vi "fitting.vi"(0 "fitting type":dbl, 5 "2D data":dbl[][](array[numeric]), 7 "force guess?":bool, 9 "force guess value":dbl[](array[numeric])) -> (4 "best fit":dbl[][](array[numeric]), 6 "best fit parameters":dbl[](array[numeric]))   [LabVIEW 2013]
uses:
  <vilib>/gmath/NumericalOptimization/Nonlinear Curve Fit LM.vi
  <vilib>/gmath/NI_Gmath.lvlib
panel:
  out "number of function calls":i32 caption="函数调用次数"
  out "数组":i32[](array[numeric])
  out "输出数组":dbl[](array[numeric])
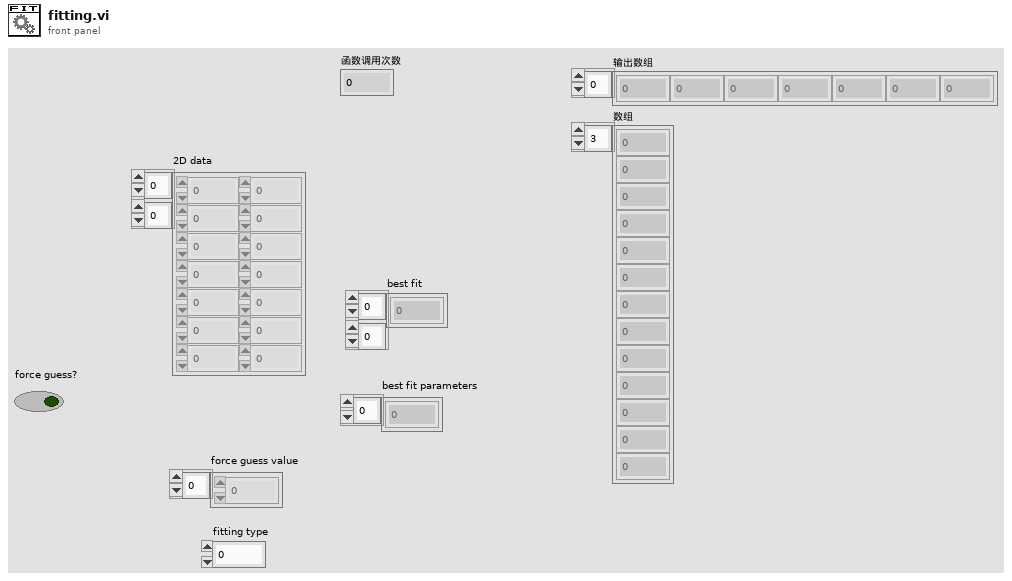
[diagram p1: front panel]
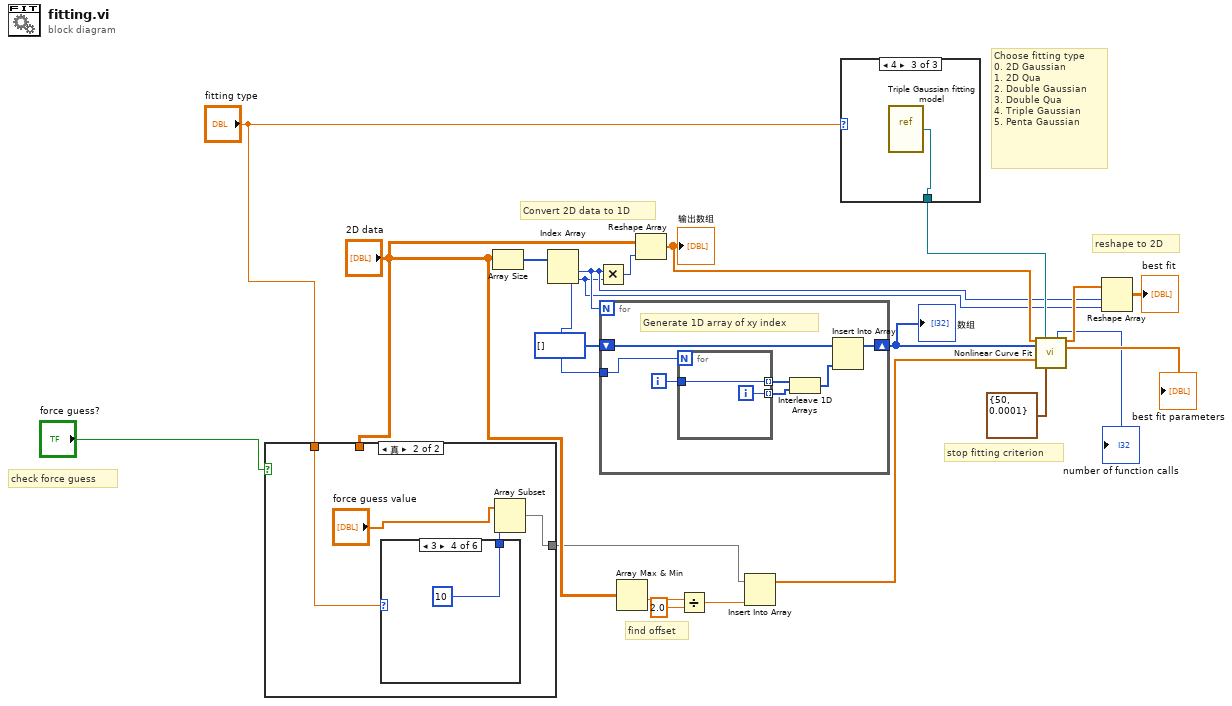
[diagram p0: block diagram]
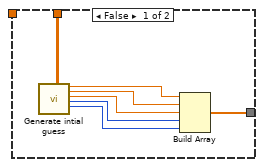
[diagram p2: hidden frame]
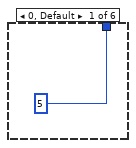
[diagram p3: hidden frame]
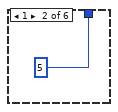
[diagram p4: hidden frame]
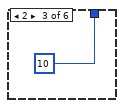
[diagram p5: hidden frame]
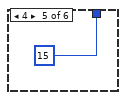
[diagram p6: hidden frame]
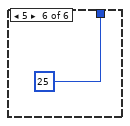
[diagram p7: hidden frame]
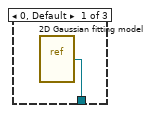
[diagram p8: hidden frame]
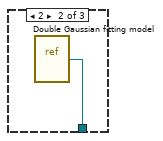
[diagram p9: hidden frame]
diagram:
  # "reshape to 2D"
  # "stop fitting criterion"
  # "find offset"
  # "check force guess"
  # "Choose fitting type\n0. 2D Gaussian\n1. 2D Qua\n2. Double Gaussian\n3. Double Qua\n4. Triple Gaussian\n5. Penta Gaussian"
  # "Convert 2D data to 1D"
  n1 = case shown="真" "force guess?" {
    tunnel: "2D data" -> [w28 _]
    tunnel: "fitting type" -> [_ w32]
    tunnel: [w22 w29] -> w10
    frame False {
      n2 = call "Generate intial guess.vi"("数组"=w28) -> ("peak"=w27:dbl, "xc"=w26:dbl, "yc"=w25:dbl, "sigx"=w24:i32, "sigy"=w23:i32)  [unwired: 14 in]
      n3 = Build Array(w27, w26, w25, w24, w23) -> (w22:dbl[])
    }
    frame True {
      n4 = case shown="3" w32 {
        tunnel: [5 ("长度") 5 ("长度") 10 ("长度") 10 ("长度") 15 ("长度") 25 ("长度")] -> w30
        frame 0, Default {
        }
        frame 1 {
        }
        frame 2 {
        }
        frame 3 {
        }
        frame 4 {
        }
        frame 5 {
        }
      }
      n5 = Array Subset(array="force guess value", length=w30) -> (w29:dbl[])  [unwired: 1 in]
    }
  }
  n6 = Array Size(array="2D data") -> (size(s)=w21:i32[])
  n7 = Index Array(array=w21) -> (element #1=w4:i32, element #2=w3:i32)  [unwired: 2 in]
  n8 = Multiply(x=w4, y=w3) -> (x*y=w20:i32)
  n9 = for {
    N: w4 -> [_]
    tunnel: w3 -> [w44]
    shift-right: [w43] -> w17
    shift-left: i32[] [] -> [w42]
    i -> [w45]
    # "Generate 1D array of xy index"
    n10 = for {
      N: w44 -> [_]
      tunnel: [w47] -> w40 mode=indexing
      tunnel: w45 -> [w47]
      tunnel: [w46] -> w39 mode=indexing
      i -> [w46]
    }
    n11 = Interleave 1D Arrays(w40, w39) -> (w41:i32[])
    n12 = Insert Into Array(array=w42, new element=w41) -> (w43:i32[])  [unwired: 1 in]
  }
  "数组" <- w17
  n13 = Array Max & Min(array="2D data") -> (min value=w12:dbl)  [unwired: 3 out]
  n14 = Reshape Array("2D data", w20) -> (w18:dbl[])
  "输出数组" <- w18
  n15 = Divide(x=w12, y=2.0) -> (x/y=w9:dbl)
  n16 = Insert Into Array(array=w10, new element=w9) -> (w8:dbl[])  [unwired: 1 in]
  n17 = case shown="4" "fitting type" {
    tunnel: [w48 w49 w50] -> w16
    frame 0, Default {
      n18 = vi-ref "2D Gaussian fitting model.vi"() -> (w48:refnum<vi>)
    }
    frame 2 {
      n19 = vi-ref "Double Gaussian fitting model.vi"() -> (w49:refnum<vi>)
    }
    frame 4 {
      n20 = vi-ref "Triple Gaussian fitting model.vi"() -> (w50:refnum<vi>)
    }
  }
  n21 = call-poly <vilib>:"Nonlinear Curve Fit.vi"("Y"=w18, "f(x,a)"=w16, "X"=w17, "initial parameters"=w8, "termination"=cluster{"max iteration":i32, "tolerance":dbl} {"max iteration"=50, "tolerance"=0.0001}) -> ("number of function calls"=→"number of function calls":i32, "best nonlinear fit"=w5:dbl[], "best fit parameters"=→"best fit parameters":dbl[])  [unwired: 5 in, 3 out]
  n22 = Reshape Array(w5, w4, w3) -> (→"best fit":dbl[][])
